vi "UTF-8 To Encoded String.vi"(8 "error in (no error)":errorcluster, 10 "UTF-8 string":string, 11 "Encoding in":refnum<class "CConfig UTF-8-BOM Encoding.lvclass">) -> (0 "error out":errorcluster, 2 "Encoded string":string, 3 "Encoding out":refnum<class "CConfig UTF-8-BOM Encoding.lvclass">)   [LabVIEW 2013, in "CConfig UTF-8-BOM Encoding.lvclass"]
doc: "Copyright 2018, Carya Automatisering, Wiebe Walstra."
uses:
  CConfig UTF-8-BOM Encoding.lvclass
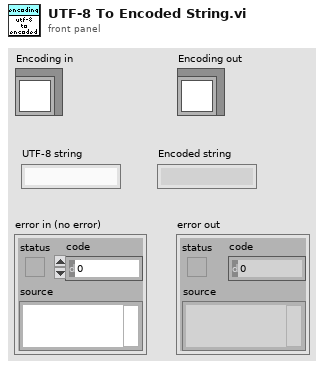
[diagram p1: front panel]
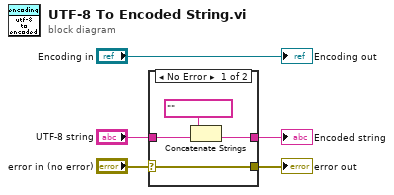
[diagram p0: block diagram]
diagram:
  n1 = case shown="No Error" "error in (no error)" {
    selector: "error in (no error)" -> [w9 w10]
    tunnel: [w9 w10] -> w3
    tunnel: "UTF-8 string" -> [w8 w11]
    tunnel: [w7 w11] -> w1
    frame No Error {
      n2 = Concatenate Strings("﻿" ("true string"), w8) -> (w7:string)
    }
    frame Error {
    }
  }
  "error out" <- w3
  "Encoded string" <- w1
  "Encoding out" <- "Encoding in"
